vi "Compile - Tx Channel Refs.vi"(6 "Packet Name":string, 7 "Timestamp Present?":bool, 8 "error in (no error)":errorcluster, 11 "Item Ref in":T1 format="%.0x") -> (0 "error out":errorcluster, 2 "Data types":T3[](array[typedef]), 3 "Item Ref out":T1 format="%.0x", 4 "Tx Ref Array":T2(array[cluster]) {"VS Refs" format="%.0x"})   [LabVIEW 2019, in "UDP-Custom-Device System Explorer.lvlib"]
uses:
  UDP-Custom-Device System Explorer.lvlib
  Shared/Types/Shared - Channel Data Type.ctl
  <vilib>/NI VeriStand/Custom Device API/Custom Device Item Ref.ctl
  Property Accessors/Tx Packet Accessors.lvlib
  <vilib>/NI VeriStand/Custom Device API/Custom Device API.lvlib
  Shared/UDP-Custom-Device Shared.lvlib
  <vilib>/NI VeriStand/Custom Device Tools/Custom Device Utility Library/Custom Device Utility Library.lvlib
  Property Accessors/Shared Packet Accessors.lvlib
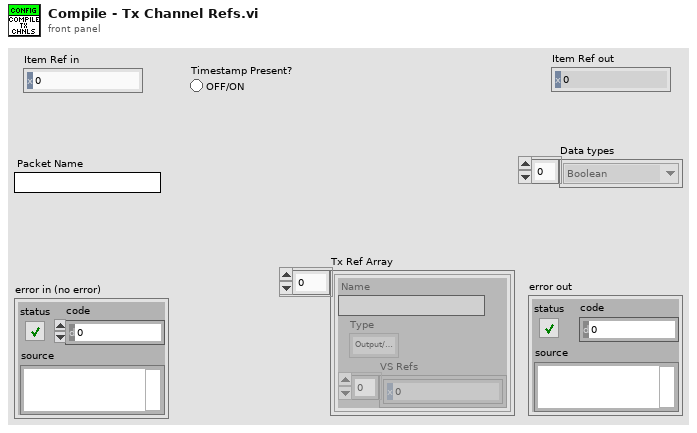
[diagram p1: front panel]
types:
  T1 = typedef "Custom Device API.lvlib/Custom Device Item Ref.ctl" = u64
  T2 = cluster{"Name":string, "Type":enum16{"Output/Write", "Input/Read", "Input/ReadWrite"}, "VS Refs":T1[]}[]
  T3 = typedef "UDP-Custom-Device Shared.lvlib/Shared - Channel Data Type.ctl" = enum16{"Boolean", "Single", "Double", "I8", "I16", "I32", "I64", "U8", "U16", "U32", "U64"}
  T4 = cluster{"Name":string, "Type":enum16{"Output/Write", "Input/Read", "Input/ReadWrite"}, "VS Refs":T1[]}
  T5 = enum16{"Output/Write", "Input/Read", "Input/ReadWrite"}
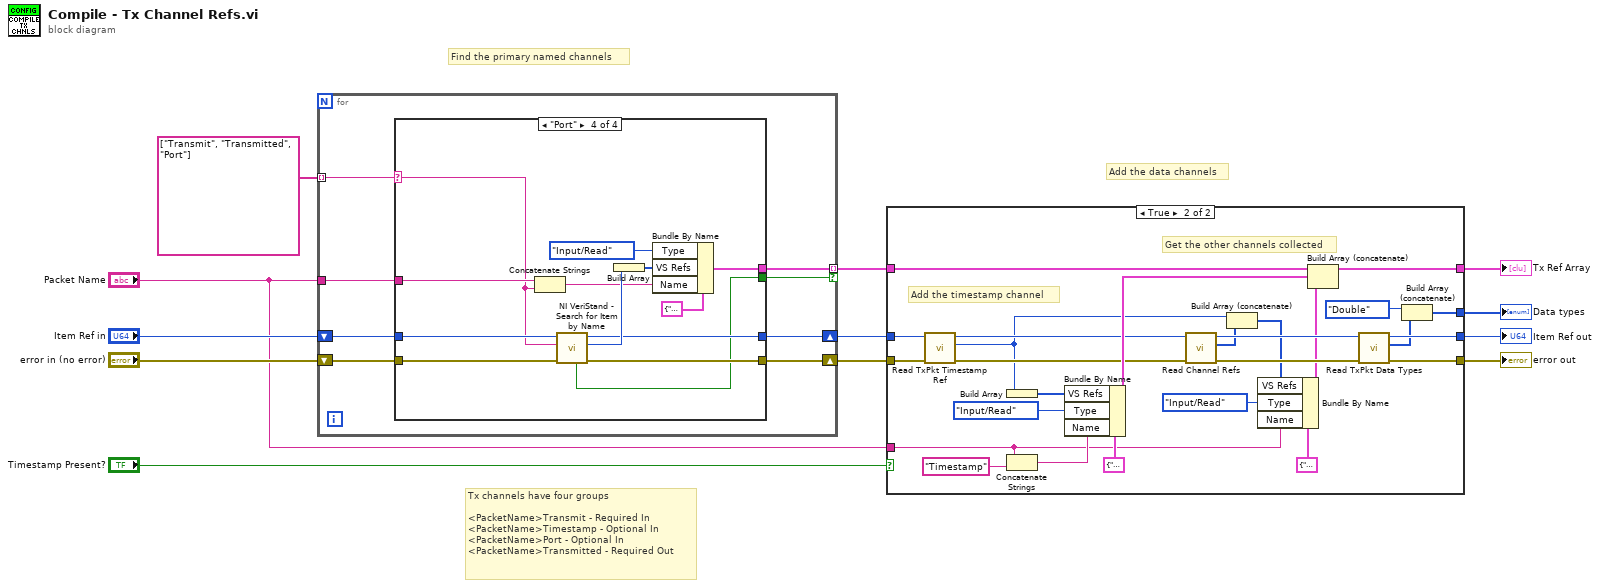
[diagram p0: block diagram]
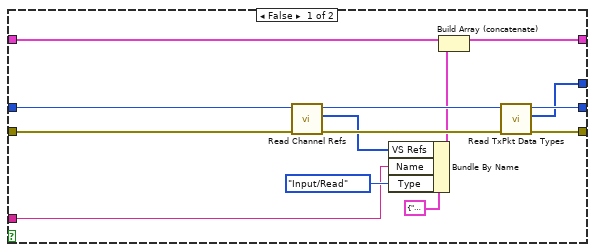
[diagram p2: hidden frame]
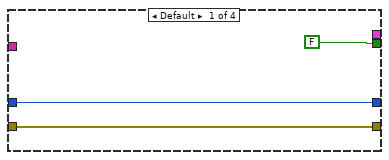
[diagram p3: hidden frame]
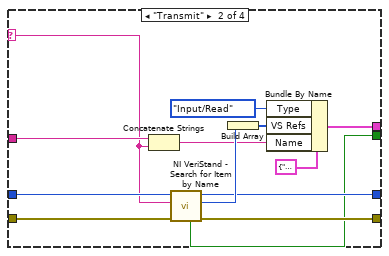
[diagram p4: hidden frame]
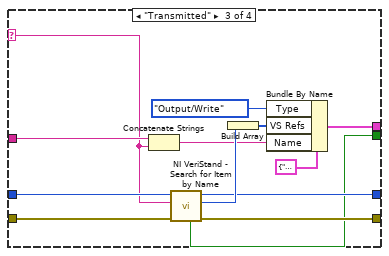
[diagram p5: hidden frame]
diagram:
  # "Add the data channels"
  # "Find the primary named channels"
  # "Tx channels have four groups\n\n<PacketName>Transmit - Required In\n<PacketName>Timestamp - Optional In\n<PacketName>Port - Optional In\n<PacketName>Transmitted - Required Out"
  n1 = for {
    tunnel: string[] ["Transmit", "Transmitted", "Port"] ("Item GUID") -> [w20] mode=indexing
    tunnel: "Packet Name" -> [w15]
    tunnel: [w17] -> w3 mode=indexing if=w16
    shift-right: [w14] -> w2
    shift-left: "Item Ref in" -> [w18]
    shift-right: [w13] -> w1
    shift-left: "error in (no error)" -> [w19]
    n2 = case shown="\"Port\"" w20 {
      selector: w20 -> [_ w25 w38 w51]
      tunnel: w19 -> [w22 w31 w44 w57]
      tunnel: w18 -> [w23 w32 w45 w58]
      tunnel: [w23 w30 w43 w56] -> w14
      tunnel: [w22 w29 w42 w55] -> w13
      tunnel: [_ w28 w41 w54] -> w17
      tunnel: [FALSE ("Found") w27 w40 w53] -> w16
      tunnel: w15 -> [_ w26 w39 w52]
      frame Default {
      }
      frame "Transmit" {
        n3 = Concatenate Strings(w26, w25) -> (w24:string)
        n4 = call <vilib>:"NI VeriStand - Search for Item by Name.vi"("error in"=w31, "Item Name"=w25, "Section Ref in"=w32) -> ("error out"=w29:errorcluster, "Item Ref"=w34:T1, "Section Ref out"=w30:T1, "Found"=w27:bool)  [unwired: 5 in]
        n5 = Build Array(w34) -> (w35:T1[])
        n6 = Bundle By Name(cluster=T4 {"Name"="", "Type"=enum."Output/Write", "VS Refs"=[]} ("Group"), "Type"=T5."Input/Read", "VS Refs"=w35, "Name"=w24) -> (w28:T4)
      }
      frame "Transmitted" {
        n7 = Concatenate Strings(w39, w38) -> (w37:string)
        n8 = call <vilib>:"NI VeriStand - Search for Item by Name.vi"("error in"=w44, "Item Name"=w38, "Section Ref in"=w45) -> ("error out"=w42:errorcluster, "Item Ref"=w47:T1, "Section Ref out"=w43:T1, "Found"=w40:bool)  [unwired: 5 in]
        n9 = Build Array(w47) -> (w48:T1[])
        n10 = Bundle By Name(cluster=T4 {"Name"="", "Type"=enum."Output/Write", "VS Refs"=[]} ("Group"), "Type"=T5."Output/Write", "VS Refs"=w48, "Name"=w37) -> (w41:T4)
      }
      frame "Port" {
        n11 = Concatenate Strings(w52, w51) -> (w50:string)
        n12 = call <vilib>:"NI VeriStand - Search for Item by Name.vi"("error in"=w57, "Item Name"=w51, "Section Ref in"=w58) -> ("error out"=w55:errorcluster, "Item Ref"=w60:T1, "Section Ref out"=w56:T1, "Found"=w53:bool)  [unwired: 5 in]
        n13 = Build Array(w60) -> (w61:T1[])
        n14 = Bundle By Name(cluster=T4 {"Name"="", "Type"=enum."Output/Write", "VS Refs"=[]} ("Group"), "Type"=T5."Input/Read", "VS Refs"=w61, "Name"=w50) -> (w54:T4)
      }
    }
  }
  n15 = case shown="True" "Timestamp Present?" {
    tunnel: w3 -> [w64 w102]
    tunnel: w2 -> [w72 w96]
    tunnel: [w75 w93] -> w5
    tunnel: [w76 w94] -> w6
    tunnel: w1 -> [w70 w95]
    tunnel: [w63 w101] -> w8
    tunnel: "Packet Name" -> [w66 w79]
    tunnel: [w74 w90] -> w12
    frame False {
      n16 = call "Read Channel Refs.vi"("error in (no error)"=w70, "Node Ptr"=w72) -> ("error out"=w69:errorcluster, "Dependent Node Refs"=w68:T1[], "Node Ptr out"=w71:T1)  [unwired: 7 in]
      n17 = Bundle By Name(cluster=T4 {"Name"="", "Type"=enum."Output/Write", "VS Refs"=[]} ("Group"), "VS Refs"=w68, "Name"=w66, "Type"=T5."Input/Read") -> (w65:T4)
      n18 = Build Array (concatenate)(w64, w65) -> (w63:T2)
      n19 = call "Read TxPkt Data Types.vi"("error in (no error)"=w69, "Node Ptr"=w71) -> ("error out"=w76:errorcluster, "Data types"=w74:T3[], "Node Ptr out"=w75:T1)  [unwired: 7 in]
    }
    frame True {
      # "Get the other channels collected"
      # "Add the timestamp channel"
      n20 = call "Read TxPkt Timestamp Ref.vi"("error in (no error)"=w95, "Node Ptr"=w96) -> ("error out"=w89:errorcluster, "Timestamp Ref"=w82:T1, "Node Ptr out"=w87:T1)  [unwired: 7 in]
      n21 = Build Array(w82) -> (w78:T1[])
      n22 = Concatenate Strings(w79, "Timestamp" ("Item GUID")) -> (w99:string)
      n23 = Bundle By Name(cluster=T4 {"Name"="", "Type"=enum."Output/Write", "VS Refs"=[]} ("Group"), "VS Refs"=w78, "Type"=T5."Input/Read", "Name"=w99) -> (w97:T4)
      n24 = call "Read Channel Refs.vi"("error in (no error)"=w89, "Node Ptr"=w87) -> ("error out"=w88:errorcluster, "Dependent Node Refs"=w84:T1[], "Node Ptr out"=w86:T1)  [unwired: 7 in]
      n25 = Build Array (concatenate)(w82, w84) -> (w83:T1[])
      n26 = Bundle By Name(cluster=T4 {"Name"="", "Type"=enum."Output/Write", "VS Refs"=[]} ("Group"), "VS Refs"=w83, "Type"=T5."Input/Read", "Name"=w79) -> (w81:T4)
      n27 = Build Array (concatenate)(w102, w97, w81) -> (w101:T2)
      n28 = call "Read TxPkt Data Types.vi"("error in (no error)"=w88, "Node Ptr"=w86) -> ("error out"=w94:errorcluster, "Data types"=w91:T3[], "Node Ptr out"=w93:T1)  [unwired: 7 in]
      n29 = Build Array (concatenate)(Shared_-_Channel_Data_Type."Double" ("element"), w91) -> (w90:T3[])
    }
  }
  "Data types" <- w12
  "Tx Ref Array" <- w8
  "error out" <- w6
  "Item Ref out" <- w5
